vi "execution class name.vi"(8 "error in":errorcluster, 11 "tag select module configuration in":refnum<class "Table Test configuration.lvclass">) -> (0 "error out":errorcluster, 2 "class name":string, 3 "tag select module configuration out":refnum<class "Table Test configuration.lvclass">)   [LabVIEW 2013, in "Table Test configuration.lvclass"]
doc: "Provides an interface for determining the module runtime class associated with this module configuration. This class name can then be used to dynamically load or locate the runtime class for initialization purposes."
uses:
  Table Test configuration.lvclass
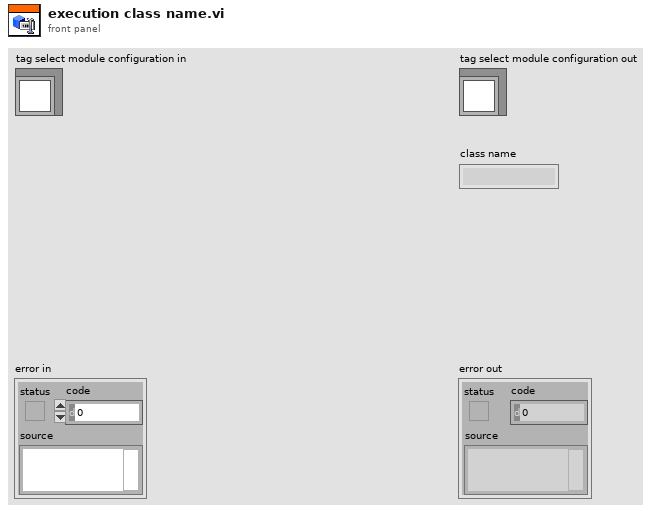
[diagram p1: front panel]
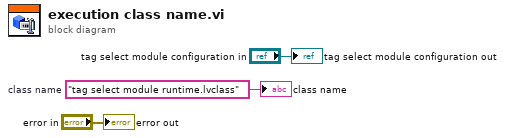
[diagram p0: block diagram]
diagram:
  w1 = "tag select module runtime.lvclass"  # class name
  "error out" <- "error in"
  "tag select module configuration out" <- "tag select module configuration in"
  "class name" <- w1
